vi "Read Record Data.vi"(8 "Error In (no error)":errorcluster, 11 "Expenses Tracker Category In":refnum<class "Expenses Tracker Category.lvclass">) -> (0 "Error Out":errorcluster, 2 "Record":variant, 3 "Expenses Tracker Category Out":refnum<class "Expenses Tracker Category.lvclass">)   [LabVIEW 2023, in "Expenses Tracker Category.lvclass"]
uses:
  Expenses Tracker Category.lvclass
  Expenses Tracker Category.lvclass/Expenses Tracker Category.ctl
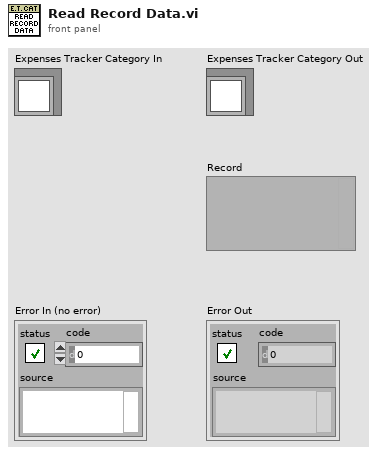
[diagram p1: front panel]
types:
  T1 = typedef "Expenses Tracker Record.lvclass/Category.ctl" = cluster{"ID":u32, "Name":string}
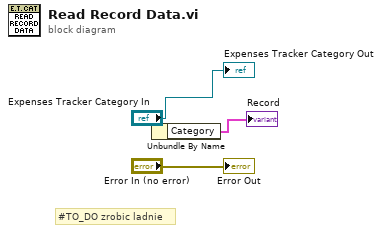
[diagram p0: block diagram]
diagram:
  # "#TO_DO zrobic ladnie"
  n1 = Unbundle By Name("Expenses Tracker Category In") -> ("Category"=→"Record":T1)
  "Error Out" <- "Error In (no error)"
  "Expenses Tracker Category Out" <- "Expenses Tracker Category In"
